vi "LVObject to JSON - Warning Input - Returns Same Warning.vi"() -> ()   [LabVIEW 2017, in "Tests.lvlib"]
uses:
  Tests.lvlib
  Flatten To JSON Object/Flatten To JSON Object.lvclass
  <vilib>/Utility/error.llb/Error Cluster From Error Code.vi
  <vilib>/addons/_JKI Toolkits/Caraya/classes/Assert/Assert Equal Value_Variant.vi
  <vilib>/ErrorRing/Error Ring.xnode
  <vilib>/addons/_JKI Toolkits/Caraya/classes/Test/Test.lvclass
  <vilib>/addons/_JKI Toolkits/Caraya/classes/Assert/Assert.lvclass
panel:
  out "error out":errorcluster
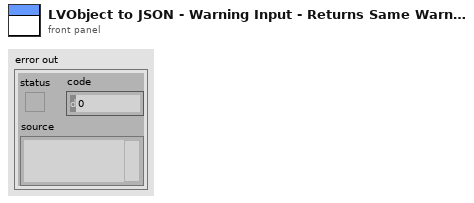
[diagram p1: front panel]
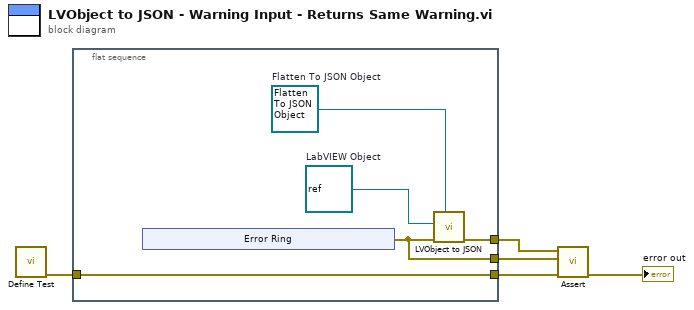
[diagram p0: block diagram]
diagram:
  n1 = call <vilib>:"Define Test.vi"() -> ("error out"=w4:errorcluster)  [unwired: 11 in]
  n2 = flat-sequence {
    tunnel: w4 -> [w8]
    tunnel: [w8] -> w3
    tunnel: [w7] -> w2
    tunnel: [w6] -> w1
    frame #0 {
      w9 = refnum<class> refnum  # LabVIEW Object
      w10 = refnum<class "Flatten To JSON Object.lvclass"> refnum  # Flatten To JSON Object
      n3 = xnode "Error Ring"() -> ("error out"=w6:errorcluster)
      n4 = call-dynamic "LVObject to JSON.vi"("Flatten To JSON Object in"=w10, "error in (no error)"=w6, "Object"=w9) -> ("error out"=w7:errorcluster)  [unwired: 7 in, 1 out]
    }
  }
  n5 = call-poly <vilib>:"Assert.vi"("error in (no error)"=w3, "Y"=w1, "X"=w2) -> ("error out"=→"error out":errorcluster)  [unwired: 8 in]
